vi "changePGAGain.vi"(8 "error in (no error)":errorcluster, 10 "Preamplifier Gain":u8 min=1, 11 "ILC in":refnum<class "ILC.lvclass">) -> (0 "error out":errorcluster, 3 "ILC out":refnum<class "ILC.lvclass">)   [LabVIEW 2013, in "ILCCommon.lvlib" / "ILC.lvclass"]
uses:
  <userlib>/Common/ILC/ILC/ILC.lvclass
  <userlib>/Common/ILC/ILC/ILC.lvclass/ILC.ctl
  <userlib>/Common/SerialProtocols/SerialCommunicator/SerialCommunicator.lvclass
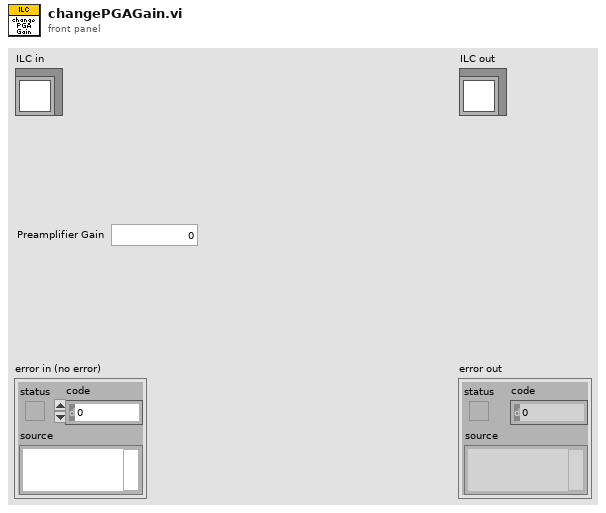
[diagram p1: front panel]
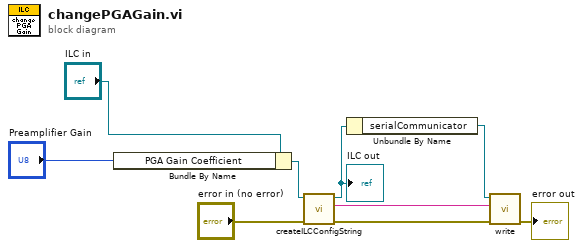
[diagram p0: block diagram]
diagram:
  n1 = Bundle By Name(cluster="ILC in", "PGA Gain Coefficient"="Preamplifier Gain") -> (w6:refnum<class "ILC.lvclass">)
  n2 = call <userlib>:"createILCConfigString.vi"("error in (no error)"="error in (no error)", "ILC in"=w6) -> ("error out"=w7:errorcluster, "ilcConfigurationString"=w8:string, "ILC out"=w4:refnum<class "ILC.lvclass">)  [unwired: 7 in]
  "ILC out" <- w4
  n3 = Unbundle By Name(w4) -> ("serialCommunicator"=w9:refnum<class "SerialCommunicator.lvclass">)
  n4 = call-dynamic "write.vi"("error in (no error)"=w7, "writeString"=w8, "SerialCommunicator in"=w9) -> ("error out"=→"error out":errorcluster)  [unwired: 7 in, 1 out]
